vi "MyQueueDriver.vi"(0 "Element To Enqueue":string, 5 "StateArray":string[](array[string]), 7 "Element To Enstack":string, 9 "name":string, 11 "error in":errorcluster, 13 "Operation":T1) -> (4 "Dequeued Element":string, 15 "error out":errorcluster)   [LabVIEW 2020]
uses:
  TypeDefs/QueueOperations.ctl
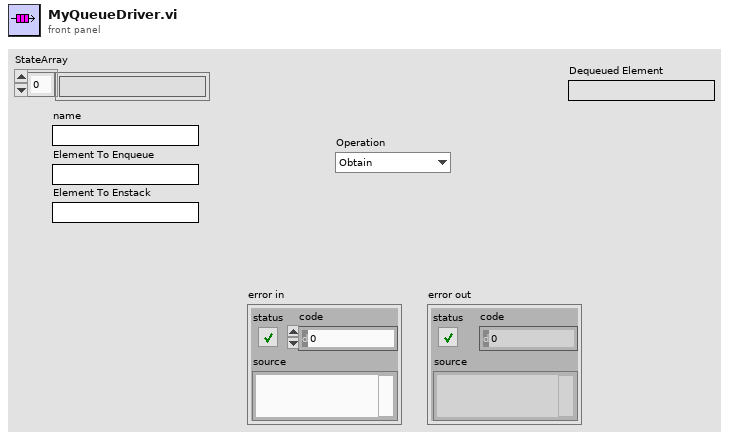
[diagram p1: front panel]
types:
  T1 = typedef "QueueOperations.ctl" = enum16{"Obtain", "Enqueue", "Enstack", "EnqueueArray", "Dequeue", "Flush", "Release"}
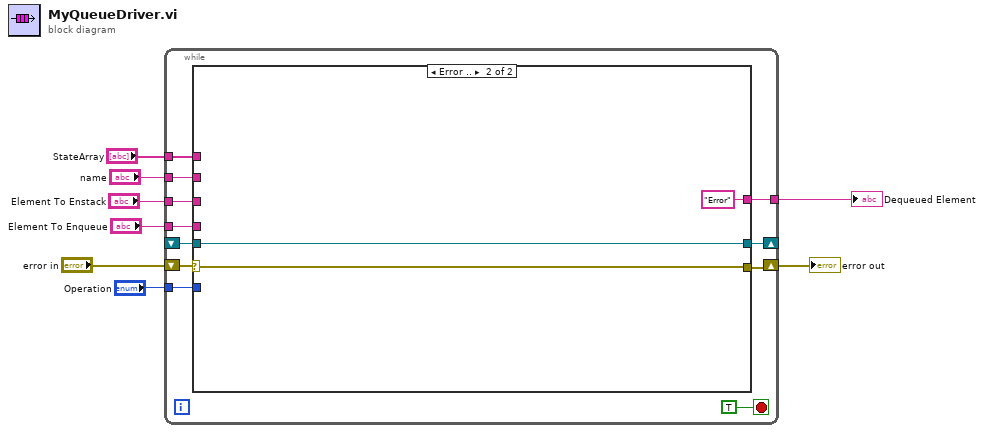
[diagram p0: block diagram]
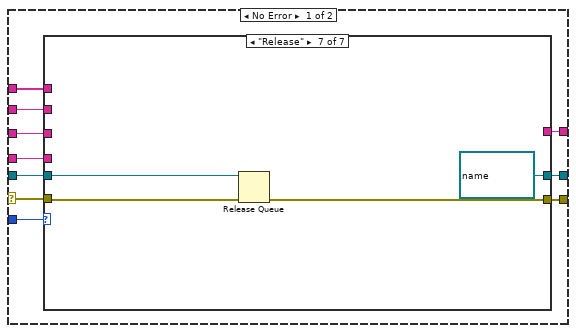
[diagram p2: hidden frame]
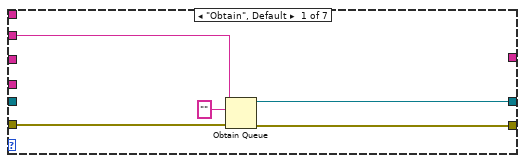
[diagram p3: hidden frame]
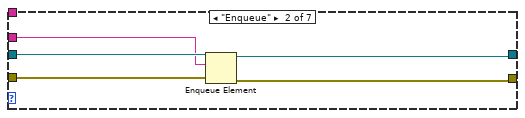
[diagram p4: hidden frame]
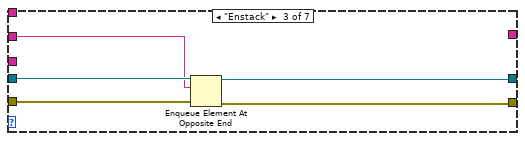
[diagram p5: hidden frame]
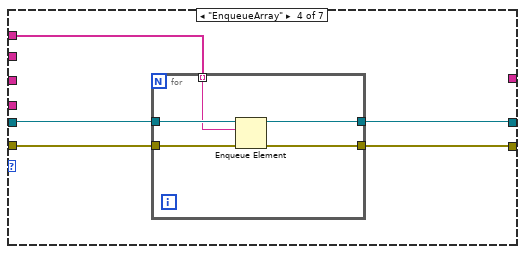
[diagram p6: hidden frame]
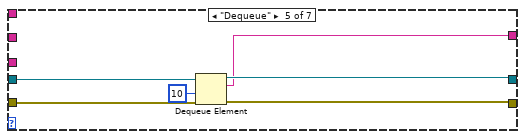
[diagram p7: hidden frame]
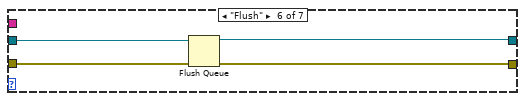
[diagram p8: hidden frame]
diagram:
  n1 = while {
    tunnel: "Operation" -> [w18]
    shift-right: [w16] -> w6
    shift-left: "error in" -> [w17]
    tunnel: "name" -> [w15]
    shift-right: [w14] -> _
    shift-left: _ -> [w13]
    tunnel: "Element To Enqueue" -> [w12]
    tunnel: "Element To Enstack" -> [w11]
    tunnel: "StateArray" -> [w10]
    tunnel: [w9] -> w1
    stop <- TRUE stop-if-true
    n2 = case shown="Error .." w17 {
      selector: w17 -> [w28 w70]
      tunnel: w18 -> [w29 _]
      tunnel: [w27 w70] -> w16
      tunnel: w15 -> [w26 _]
      tunnel: [w25 w71] -> w14
      tunnel: w13 -> [w24 w71]
      tunnel: w12 -> [w23 _]
      tunnel: w11 -> [w22 _]
      tunnel: w10 -> [w21 _]
      tunnel: [w20 "Error" ("name")] -> w9
      frame No Error {
        n3 = case shown="\"Release\"" w29 {
          tunnel: w28 -> [w34 w39 w44 w49 w60 w64 w68]
          tunnel: [w33 w38 w43 w48 w59 w63 w67] -> w27
          tunnel: w26 -> [w32 _ _ _ _ _ _]
          tunnel: [w30 w37 w42 w47 w57 w62 refnum<queue> refnum ("queue out")] -> w25
          tunnel: w24 -> [_ w36 w41 w46 w58 w61 w65]
          tunnel: w23 -> [_ w35 _ _ _ _ _]
          tunnel: w22 -> [_ _ w40 _ _ _ _]
          tunnel: w21 -> [_ _ _ w45 _ _ _]
          tunnel: [_ _ _ _ w55 _ _] -> w20
          frame "Obtain", Default {
            n4 = Obtain Queue(name (unnamed)=w32, element data type="" ("name"), error in (no error)=w34) -> (queue out=w30:refnum<queue>, error out=w33:errorcluster)  [unwired: 2 in, 1 out]
          }
          frame "Enqueue" {
            n5 = Enqueue Element(queue=w36, element=w35, error in (no error)=w39) -> (queue out=w37:refnum<queue>, error out=w38:errorcluster)  [unwired: 1 in, 1 out]
          }
          frame "Enstack" {
            n6 = Enqueue Element At Opposite End(queue=w41, element=w40, error in (no error)=w44) -> (queue out=w42:refnum<queue>, error out=w43:errorcluster)  [unwired: 1 in, 1 out]
          }
          frame "EnqueueArray" {
            n7 = for {
              tunnel: w49 -> [w54]
              tunnel: [w53] -> w48
              tunnel: [w52] -> w47
              tunnel: w46 -> [w51]
              tunnel: w45 -> [w50] mode=indexing
              n8 = Enqueue Element(queue=w51, element=w50, error in (no error)=w54) -> (queue out=w52:refnum<queue>, error out=w53:errorcluster)  [unwired: 1 in, 1 out]
            }
          }
          frame "Dequeue" {
            n9 = Dequeue Element(queue=w58, timeout in ms (-1)=10, error in (no error)=w60) -> (queue out=w57:refnum<queue>, element=w55:string, error out=w59:errorcluster)  [unwired: 1 out]
          }
          frame "Flush" {
            n10 = Flush Queue(queue=w61, error in (no error)=w64) -> (queue out=w62:refnum<queue>, error out=w63:errorcluster)  [unwired: 1 out]
          }
          frame "Release" {
            n11 = Release Queue(queue=w65, error in (no error)=w68) -> (error out=w67:errorcluster)  [unwired: 1 in, 2 out]
          }
        }
      }
      frame Error {
      }
    }
  }
  "error out" <- w6
  "Dequeued Element" <- w1
